vi "HVPPS FGV Ref.vi"(6 "Option":T1, 8 "error in":errorcluster, 10 "Socket No":u16, 11 "PowerSupplyIn.lvclass":refnum<class "PowerSupply.lvclass">) -> (0 "error out":errorcluster, 3 "PowerSupplyOut.lvclass":refnum<class "PowerSupply.lvclass">)   [LabVIEW 2023, in "HardwareAbstractionLayer_LVOOP.lvlib" / "PowerSupply.lvclass"]
uses:
  PowerSupply.lvclass
  Control/PPS FGV Option.ctl
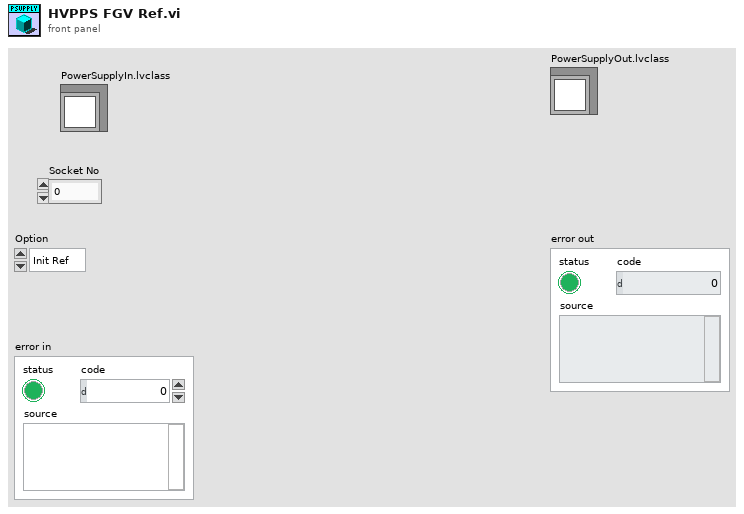
[diagram p1: front panel]
types:
  T1 = typedef "HardwareAbstractionLayer_LVOOP.lvlib/PowerSupply.lvclass/PPS FGV Option.ctl" = enum16{"Init Ref", "Get Ref", "Set Ref"}
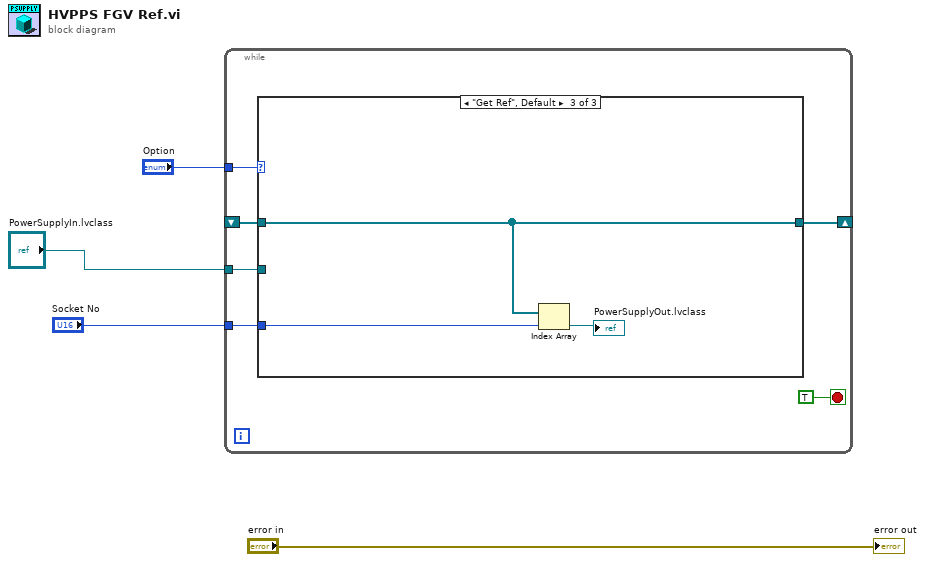
[diagram p0: block diagram]
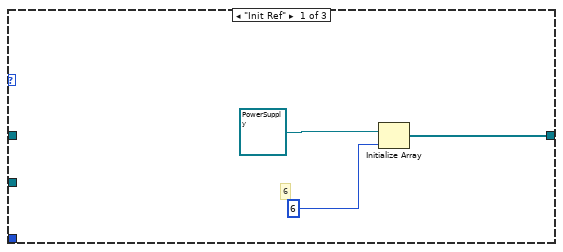
[diagram p2: hidden frame]
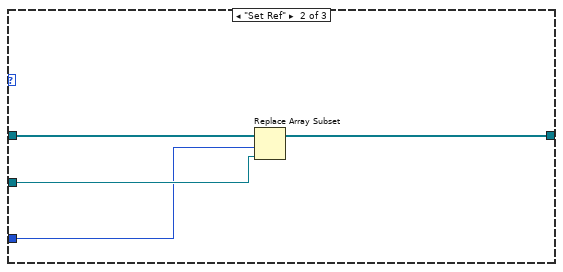
[diagram p3: hidden frame]
diagram:
  n1 = while {
    tunnel: "Option" -> [w9]
    shift-right: [w8] -> _
    shift-left: _ -> [w7]
    tunnel: "PowerSupplyIn.lvclass" -> [w6]
    tunnel: "Socket No" -> [w5]
    stop <- TRUE stop-if-true
    n2 = case shown="\"Get Ref\", Default" w9 {
      tunnel: [w12 w16 w20] -> w8
      tunnel: w7 -> [_ w17 w20]
      tunnel: w6 -> [_ w15 _]
      tunnel: w5 -> [_ w14 w19]
      frame "Init Ref" {
        # "6"
        n3 = Initialize Array(refnum<class "PowerSupply.lvclass"> refnum ("HardwareAbstractionLayer_LVOOP.lvlib:PowerSupply.lvclass"), 6 ("dimension size")) -> (w12:refnum<class "PowerSupply.lvclass">[])
      }
      frame "Set Ref" {
        n4 = Replace Array Subset(array=w17, new element=w15, index=w14) -> (w16:refnum<class "PowerSupply.lvclass">[])
      }
      frame "Get Ref", Default {
        n5 = Index Array(array=w20, index=w19) -> (element=→"PowerSupplyOut.lvclass":refnum<class "PowerSupply.lvclass">)
      }
    }
  }
  "error out" <- "error in"
